vi "VISA_Communication.vi"(8 "error in (no error)":errorcluster, 10 "baud rate (9600)":u32=9600, 11 "VISA Refnum in":refnum<visa-resource-name>) -> (0 "error out":errorcluster, 3 "VISA Refnum out":refnum<visa-resource-name>)   [LabVIEW 2026]
uses:
  <vilib>/Instr/_visa.llb/VISA Configure Serial Port (Instr).vi
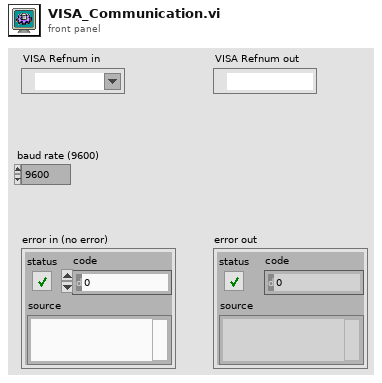
[diagram p1: front panel]
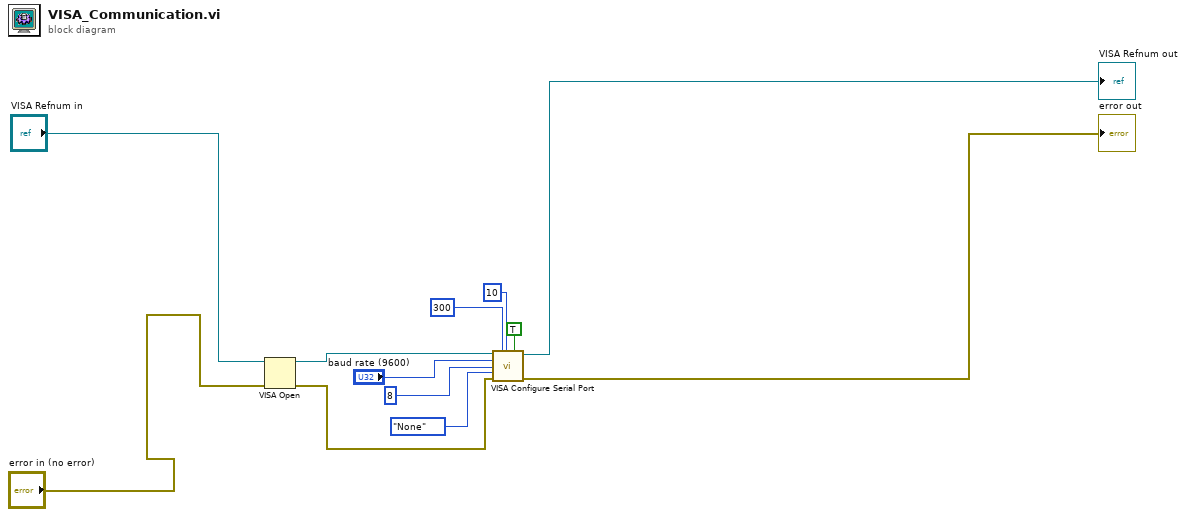
[diagram p0: block diagram]
diagram:
  n1 = VISA Open(error in (no error)="error in (no error)", VISA resource name="VISA Refnum in") -> (VISA resource name=w3:refnum<visa-resource-name>, error out=w1:errorcluster)  [unwired: 3 in]
  n2 = call-poly "VISA Configure Serial Port"("VISA resource name"=w3, "timeout (10sec)"=u32 300, "termination char\n(0xA = '\\n' = LF)"=u32 10 ("timeout (10sec)"), "Enable Termination\nChar (T)"=TRUE ("Enable Termination\nChar (T)"), "baud rate (9600)"="baud rate (9600)", "data bits (8)"=u16 8, "parity (0:none)"=enum16{"None", "Odd", "Even", "Mark", "Space"}."None", "error in (no error)"=w1) -> ("VISA resource name out"=→"VISA Refnum out":refnum<visa-resource-name>, "error out"=→"error out":errorcluster)  [unwired: 6 in]
